vi "SetParam.vi"(8 "error in (no error)":errorcluster caption="entrée d'erreur (pas d'erreur)", 10 "GroupKFold":cluster{"n_splits":i32}={"n_splits"=5}, 11 "GroupKFold.lvclass":refnum<class "GroupKFold.lvclass">) -> (0 "error out":errorcluster caption="sortie d'erreur", 3 "GroupKFold.lvclass":refnum<class "GroupKFold.lvclass">)   [LabVIEW 2020, in "GroupKFold.lvclass"]
doc: "Set Parameters"
uses:
  GroupKFold.lvclass
  GroupKFold.lvclass/GroupKFold.ctl
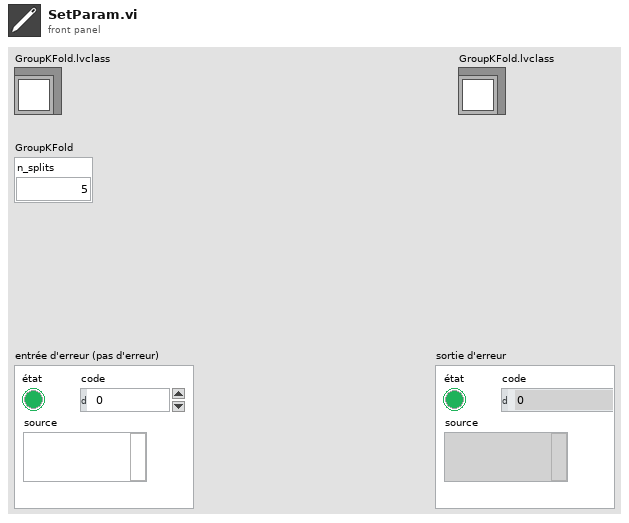
[diagram p1: front panel]
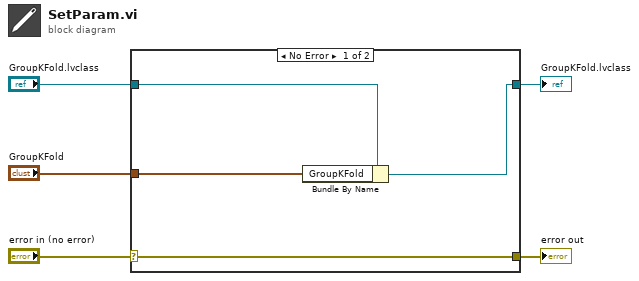
[diagram p0: block diagram]
diagram:
  n1 = case shown="No Error" "error in (no error)" {
    selector: "error in (no error)" -> [w9 w10]
    tunnel: [w9 w10] -> w4
    tunnel: [w7 w11] -> w2
    tunnel: "GroupKFold.lvclass" -> [w8 w11]
    tunnel: "GroupKFold" -> [w6 _]
    frame No Error {
      n2 = Bundle By Name(cluster=w8, "GroupKFold"=w6) -> (w7:refnum<class "GroupKFold.lvclass">)
    }
    frame Error {
    }
  }
  "error out" <- w4
  "GroupKFold.lvclass" <- w2
